vi "Read Matlab Params.vi"(8 "error in (no error)":errorcluster, 10 "Enum":T1(ring), 11 "TrialBasedExperiment in":refnum<class "MatlabExperiment.lvclass">) -> (0 "error out":errorcluster, 2 "Matlab Param Array":cluster{"Name":string, "Data":variant}[](array[cluster]), 3 "TrialBasedExperiment out":refnum<class "MatlabExperiment.lvclass">)   [LabVIEW 2014, in "AcquisitionCoreObjects.lvlib" / "MatlabExperiment.lvclass"]
uses:
  MatlabExperiment.lvclass
  Matlab API/Matlab API.lvlib
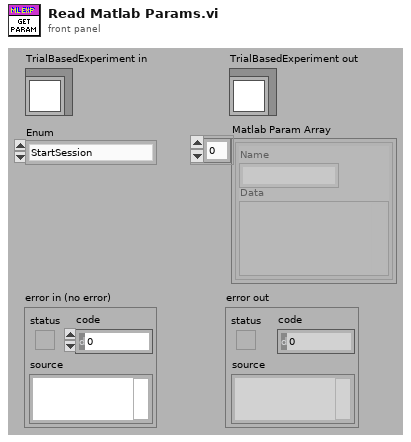
[diagram p1: front panel]
types:
  T1 = enum16{"StartSession", "StartTrial", "ShowStimulus"}
  T2 = cluster{"Name":string, "Type":string, "value":string}[]
  T3 = cluster{"Intertrial":dbl, "AcquireFixation":dbl, "HoldFixation":dbl, "DelayPeriod":dbl, "ResponsePeriod":dbl}
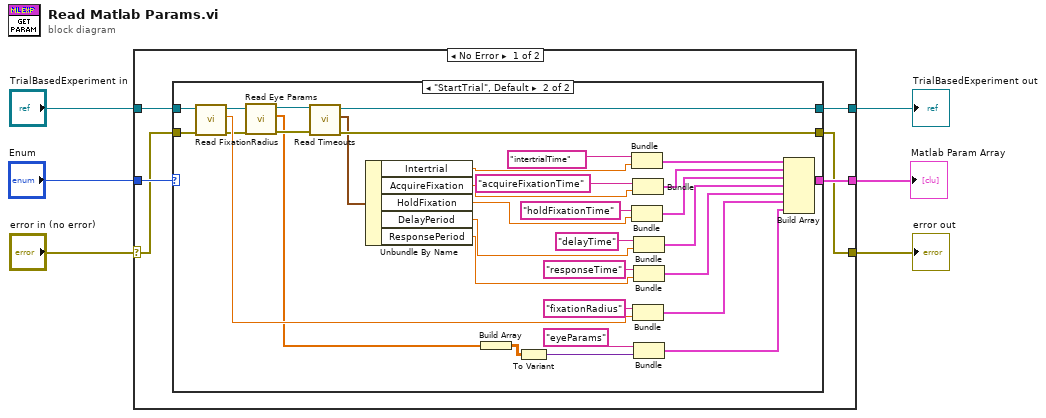
[diagram p0: block diagram]
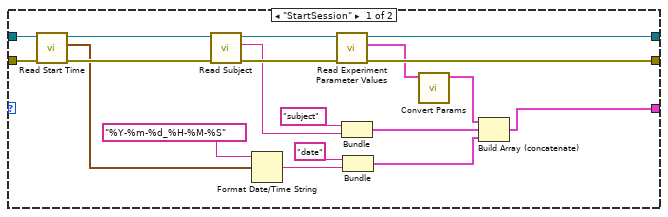
[diagram p2: hidden frame]
diagram:
  n1 = case shown="No Error" "error in (no error)" {
    selector: "error in (no error)" -> [w8 w66]
    tunnel: [w7 w66] -> w5
    tunnel: [w11 w65] -> w3
    tunnel: "TrialBasedExperiment in" -> [w10 w65]
    tunnel: "Enum" -> [w12 _]
    tunnel: [w9 _] -> w1
    frame No Error {
      n2 = case shown="\"StartTrial\", Default" w12 {
        tunnel: [w31 w48] -> w11
        tunnel: w10 -> [w19 w45]
        tunnel: [w22 w46] -> w9
        tunnel: w8 -> [w17 w44]
        tunnel: [w30 w49] -> w7
        frame "StartSession" {
          n3 = call-dynamic "Read Start Time.vi"("error in (no error)"=w17, "AcquistionObject in"=w19) -> ("error out"=w16:errorcluster, "Start Time"=w14:timestamp, "AcquistionObject out"=w18:refnum<class "MatlabExperiment.lvclass">)  [unwired: 7 in]
          n4 = call-dynamic "Read Subject.vi"("error in (no error)"=w16, "TrialBasedExperiment in"=w18) -> ("error out"=w29:errorcluster, "Subject"=w26:string, "TrialBasedExperiment out"=w28:refnum<class "MatlabExperiment.lvclass">)  [unwired: 7 in]
          n5 = Format Date/Time String(time format string (%c)="%Y-%m-%d_%H-%M-%S", seconds (now)=w14) -> (date/time string=w13:string)  [unwired: 1 in]
          n6 = call-dynamic "Read Experiment Parameter Values.vi"("error in (no error)"=w29, "TrialBasedExperiment in"=w28) -> ("error out"=w30:errorcluster, "Experiment Parameter Values"=w25:T2, "TrialBasedExperiment out"=w31:refnum<class "MatlabExperiment.lvclass">)  [unwired: 7 in]
          n7 = Bundle("subject", "Subject"=w26) -> (w24:cluster{string, "Subject":string})  [unwired: 1 in]
          n8 = Bundle("date", "date/time string"=w13) -> (w20:cluster{string, "date/time string":string})  [unwired: 1 in]
          n9 = call "Convert Params.vi"("Experiment Parameter Values"=w25) -> ("Matlab Param Array"=w23:cluster{"Name":string, "Data":variant}[])  [unwired: 10 in]
          n10 = Build Array (concatenate)(w23, w24, w20) -> (w22:cluster{"Name":string, "Data":variant}[])
        }
        frame "StartTrial", Default {
          n11 = call-dynamic "Read FixationRadius.vi"("error in (no error)"=w44, "MatlabExperiment in"=w45) -> ("error out"=w38:errorcluster, "FixationRadius"=w42:dbl, "MatlabExperiment out"=w40:refnum<class "MatlabExperiment.lvclass">)  [unwired: 7 in]
          n12 = call-dynamic "Read Eye Params.vi"("error in (no error)"=w38, "TrialBasedExperiment in"=w40) -> ("error out"=w37:errorcluster, "Eye Params"=w34:dbl[], "TrialBasedExperiment out"=w39:refnum<class "MatlabExperiment.lvclass">)  [unwired: 7 in]
          n13 = call-dynamic "Read Timeouts.vi"("error in (no error)"=w37, "TrialBasedExperiment in"=w39) -> ("error out"=w49:errorcluster, "Timeouts"=w47:T3, "TrialBasedExperiment out"=w48:refnum<class "MatlabExperiment.lvclass">)  [unwired: 7 in]
          n14 = Unbundle By Name(w47) -> ("Intertrial"=w56:dbl, "AcquireFixation"=w55:dbl, "HoldFixation"=w54:dbl, "DelayPeriod"=w53:dbl, "ResponsePeriod"=w52:dbl)
          n15 = Build Array(w34) -> (w35:dbl[][])
          n16 = To Variant(anything=w35) -> (Variant=w33:variant)
          n17 = Bundle("intertrialTime", "Intertrial"=w56) -> (w60:cluster{string, "Intertrial":dbl})  [unwired: 1 out]
          n18 = Bundle("holdFixationTime", "HoldFixation"=w54) -> (w58:cluster{string, "HoldFixation":dbl})  [unwired: 1 out]
          n19 = Bundle("acquireFixationTime", "AcquireFixation"=w55) -> (w59:cluster{string, "AcquireFixation":dbl})  [unwired: 1 out]
          n20 = Bundle("fixationRadius", "FixationRadius"=w42) -> (w41:cluster{string, "FixationRadius":dbl})  [unwired: 1 out]
          n21 = Bundle("delayTime", "DelayPeriod"=w53) -> (w51:cluster{string, "DelayPeriod":dbl})  [unwired: 1 out]
          n22 = Bundle("responseTime", "ResponsePeriod"=w52) -> (w50:cluster{string, "ResponsePeriod":dbl})  [unwired: 1 out]
          n23 = Bundle("eyeParams", "Variant"=w33) -> (w32:cluster{string, "Variant":variant})  [unwired: 1 out]
          n24 = Build Array(w60, w59, w58, w51, w50, w41, w32) -> (w46:cluster{string, "Variant":variant}[])
        }
      }
    }
    frame Error {
    }
  }
  "error out" <- w5
  "TrialBasedExperiment out" <- w3
  "Matlab Param Array" <- w1
